vi "GDSLvClass_ChangeConnectorPane.vi"(0 "ClassRefIn":refnum<vi>, 1 "ForceResaving(False)":bool, 5 "error in":errorcluster) -> (14 "ClassRefOut":refnum<vi>, 19 "error out":errorcluster)   [LabVIEW 2020]
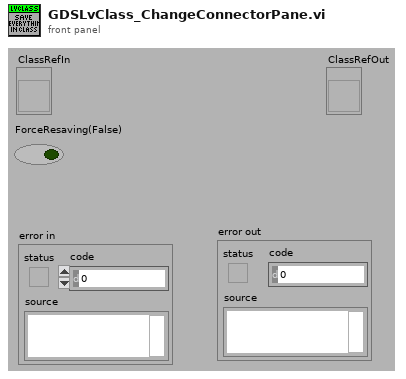
[diagram p1: front panel]
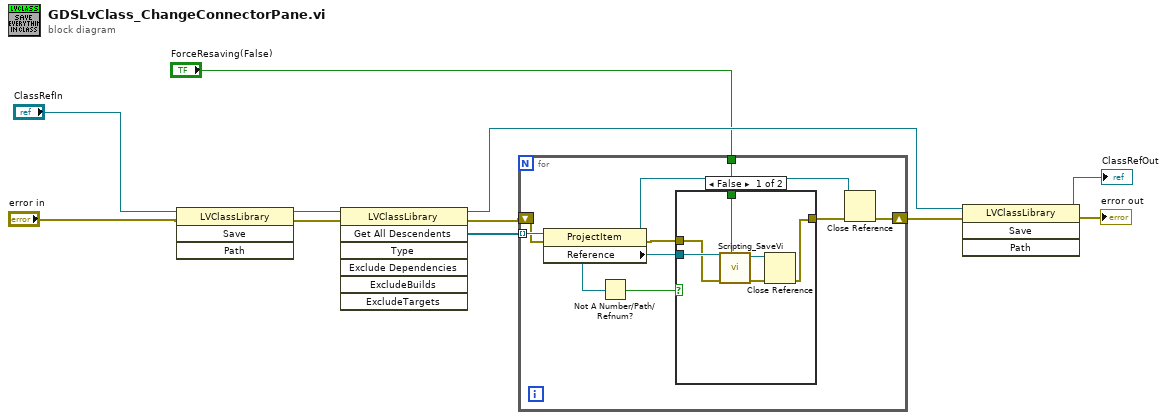
[diagram p0: block diagram]
diagram:
  n1 = invoke class="LVClassLibrary" method="Save"(reference="ClassRefIn", error in="error in") -> (reference out=w9:refnum<vi>, error out=w8:errorcluster)  [unwired: 2 in, 2 out]
  n2 = invoke class="LVClassLibrary" method="Get All Descendents"(reference=w9, error in=w8) -> (reference out=w4:refnum<vi>, error out=w6:errorcluster, "All Descendents"=w7:refnum<vi>[])  [unwired: 5 in, 4 out]
  n3 = for {
    tunnel: w7 -> [w20] mode=indexing
    shift-right: [w13] -> w5
    shift-left: w6 -> [w16]
    tunnel: "ForceResaving(False)" -> [w15]
    n4 = property class="ProjectItem"(reference=w20, error in=w16) -> (reference out=w12:refnum<vi>, error out=w17:errorcluster, "Reference"=w18:refnum<vi>)
    n5 = Not A Number/Path/Refnum?(number/path/refnum=w18) -> (NaN/Path/Refnum?=w19:bool)
    n6 = case shown="False" w19 {
      tunnel: w18 -> [w26 _]
      tunnel: w17 -> [w25 w27]
      tunnel: [w22 w27] -> w14
      tunnel: w15 -> [w21 _]
      frame False {
        n7 = call <resource>:"Scripting_SaveVi.vi"("ForceResaving(False)"=w21, "error in (no error)"=w25, "VIRefToSaveIn"=w26) -> ("error out"=w24:errorcluster, "VIRefToSaveOut"=w23:refnum<vi>)  [unwired: 7 in]
        n8 = Close Reference(reference=w23, error in (no error)=w24) -> (error out=w22:errorcluster)
      }
      frame True {
      }
    }
    n9 = Close Reference(reference=w12, error in (no error)=w14) -> (error out=w13:errorcluster)
  }
  n10 = invoke class="LVClassLibrary" method="Save"(reference=w4, error in=w5) -> (reference out=→"ClassRefOut":refnum<vi>, error out=→"error out":errorcluster)  [unwired: 2 in, 2 out]
